vi "PID Denominator.vi"(11 "Enum":T1) -> (3 "DSM Message":string)   [LabVIEW 2016]
uses:
  Custom Pallet Controls/Custom Pallet Forward.ctl
  Type Definitions/GEA2 Commands.ctl
  LabVIEW GEA2 Toolkit v1.0.0.0/library/GEA2_Toolkit.lvlib
panel:
  in  "PID Denominator":u16
  out "Description":string="Set PID Denominator Over Threshold"
  in  "Complete":T2
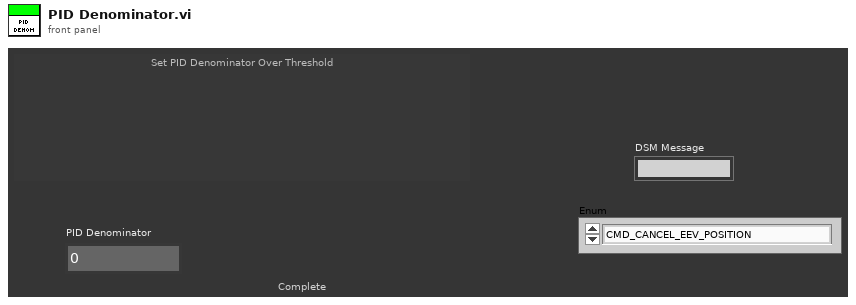
[diagram p1: front panel]
types:
  T1 = typedef "GEA2 Commands.ctl" = enum16{"CMD_CANCEL_EEV_POSITION", "CMD_CLEAR_ENERGY_USAGE_CTRS", "CMD_CLEAR_FAULT_COUNTS", "CMD_CLEAR_OVERRIDE_STATUS", "CMD_COMP_OFF", "CMD_COMP_ON", "CMD_DSM_OVERRIDES", "CMD_EEV_POSITION", "CMD_ENTER_EXIT_FCT_MODE", "CMD_ENTER_FACT_MODE", "CMD_HP_RUN_6MIN", "CMD_INITIATE_REMOTE_DSM_OVERRIDE", "CMD_LE_2_SECONDS", "CMD_REFRESH_SERVICE_TIMEOUTS", "CMD_RESET", "CMD_RESET_FILTER_TIMES", "CMD_RESTORE_EEPROM_DEFAULTS", "CMD_RQST_LED_STATUS", "CMD_SET_AMBIENT_THRESH_1", "CMD_SET_AMBIENT_THRESH_2", "CMD_SET_AMBIENT_THRESH_3", "CMD_SET_CURRENTS", "CMD_SET_EEV_DRIVE_LINES", "CMD_SET_EEV_STOP_POSITION", "CMD_SET_LEDS", "CMD_SET_MODEL_NUMBER", "CMD_SET_PID_I_DENOM_OVER_THR", "CMD_SET_PID_I_DENOM_UNDER_THR", "CMD_SET_PID_LOW_SH_TARGET", "CMD_SET_PID_MID_SH_TARGET", "CMD_SET_PID_P_DENOMINATOR", "CMD_SET_SERIAL_NUMBER", "CMD_SET_START_POS_OVER_THR", "CMD_SET_START_POS_UNDER_THR", "CMD_TOGGLE_FAN", "CMD_TOGGLE_LE_SERV", "CMD_TOGGLE_SERVICE_MODE", "CMD_TOGGLE_UE_SERV", "CMD_TURN_ON_OFF_DLB", "CMD_UE_2_SECONDS", "CMD_UPDATE_DSM_LEVEL", "CMD_UPDATE_MODE", "CMD_WRITE_SETPOINTS", "REQ_READ_KEY_STATUS", "REQ_SYSTEM_MODE", "RQST_CURRENT_PID_SH_TARGET", "RQST_DATA_FROM_DATA_FLASH", "RQST_DATA_FROM_MEMORY", "RQST_DSM_OVERRIDE_STATUS", "RQST_HEM_KWH_DATA", "RQST_HYPERTERM_OUTPUT_DATA", "RQST_IDLB_RESISTANCE", "RQST_MODEL_NUMBER", "RQST_MODEL_SELECT_AD_VALUE", "RQST_OTHER_FAULT_COUNTS", "RQST_OVERRIDE_STATUS", "RQST_PID_PARAMETERS", "RQST_READ_PERSONALITY", "RQST_SERIAL_NUMBER", "RQST_SERVICE_ERROR_CODES", "RQST_Software_Version", "RQST_SS_FAULT_COUNTS", "RQST_STATUS_QUERY", "RQST_STD_ELEC_RANGE", "RQST_SUPPORTED_MODES", "RQST_T2_RESISTANCE", "RQST_T3B_RESISTANCE", "RQST_T4_RESISTANCE", "RQST_T5_RESISTANCE", "RQST_TEMP_RANGE", "RQST_VACATION_RANGE", "RQST_WATER_CAPACITY"}
  T2 = typedef "Custom Pallet Forward.ctl" = bool
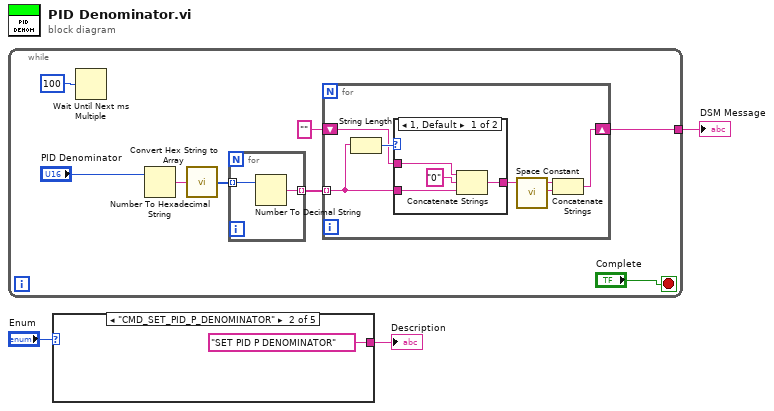
[diagram p0: block diagram]
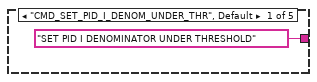
[diagram p2: hidden frame]
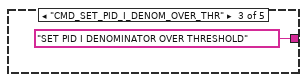
[diagram p3: hidden frame]
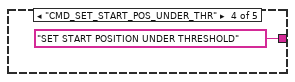
[diagram p4: hidden frame]
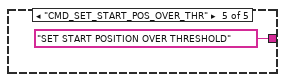
[diagram p5: hidden frame]
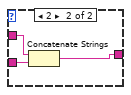
[diagram p6: hidden frame]
diagram:
  n1 = while {
    tunnel: [w6] -> w3
    stop <- "Complete" stop-if-true
    n2 = Wait Until Next ms Multiple(millisecond multiple=u32 100) -> ()  [unwired: 1 out]
    n3 = Number To Hexadecimal String(2:"PID Denominator") -> (0:w8:string)  [unwired: 1 in]
    n4 = call "Convert Hex String to Array.vi"("Hex String In"=w8) -> ("Hex Array Out"=w5:u8[])  [unwired: 14 in]
    n5 = for {
      tunnel: w5 -> [w13] mode=indexing
      tunnel: [w12] -> w4 mode=indexing
      n6 = Number To Decimal String(number=w13) -> (decimal integer string=w12:string)  [unwired: 1 in]
    }
    n7 = for {
      tunnel: w4 -> [w17] mode=indexing
      shift-right: [w14] -> w6
      shift-left: "" -> [w18]
      n8 = String Length(string=w17) -> (length=w19:i32)
      n9 = case shown="1, Default" w19 {
        tunnel: w18 -> [w23 w26]
        tunnel: [w20 w25] -> w15
        tunnel: w17 -> [w21 w24]
        frame 1, Default {
          n10 = Concatenate Strings(w23, "0" ("string"), w21) -> (w20:string)
        }
        frame 2 {
          n11 = Concatenate Strings(w26, w24) -> (w25:string)
        }
      }
      n12 = call <vilib>:"Space Constant.vi"() -> ("String"=w16:string)
      n13 = Concatenate Strings(w15, w16) -> (w14:string)
    }
  }
  "DSM Message" <- w3
  n14 = case shown="\"CMD_SET_PID_P_DENOMINATOR\"" "Enum" {
    tunnel: ["SET PID I DENOMINATOR UNDER THRESHOLD" "SET PID P DENOMINATOR" "SET PID I DENOMINATOR OVER THRESHOLD" "SET START POSITION UNDER THRESHOLD" "SET START POSITION OVER THRESHOLD"] -> w1
    frame "CMD_SET_PID_I_DENOM_UNDER_THR", Default {
    }
    frame "CMD_SET_PID_P_DENOMINATOR" {
    }
    frame "CMD_SET_PID_I_DENOM_OVER_THR" {
    }
    frame "CMD_SET_START_POS_UNDER_THR" {
    }
    frame "CMD_SET_START_POS_OVER_THR" {
    }
  }
  "Description" <- w1
